vi "reserve.vi"(7 "LabVIEW Web Service Request":refnum<class "Web Request.lvclass">, 11 "context_id":string) -> (2 "reservation_id":string, 3 "load_url":string)   [LabVIEW 2013]
uses:
  <vilib>/wsapi/Web Request.lvclass
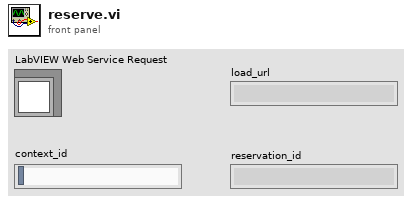
[diagram p1: front panel]
types:
  T1 = cluster{"laboratory_id":string, "username":string, "institution":string, "general_configuration_str":string, "particular_configurations":string, "request_payload":string, "user_properties":string, "locale":string, "back":string}
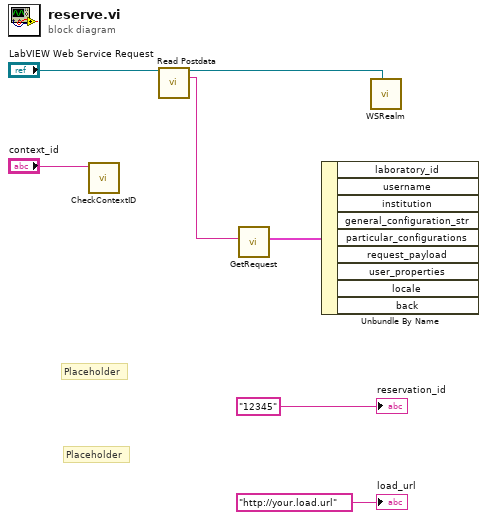
[diagram p0: block diagram]
diagram:
  # "Placeholder"
  # "Placeholder"
  n1 = call "CheckContextID.vi"("context_id"="context_id") -> ()  [unwired: 10 in, 1 out]
  n2 = call <vilib>:"Read Postdata.vi"("LabVIEW Web Service Request"="LabVIEW Web Service Request") -> ("LabVIEW Web Service Request out"=w5:refnum<class "Web Request.lvclass">, "postdata"=w4:string)  [unwired: 12 in, 1 out]
  n3 = call "GetRequest.vi"("JSON string"=w4) -> ("request"=w3:T1)  [unwired: 10 in]
  n4 = Unbundle By Name(w3) -> ()  [unwired: 9 out]
  n5 = call "WSRealm.vi"("LabVIEW Web Service Request"=w5) -> ()  [unwired: 11 in]
  "reservation_id" <- "12345"
  "load_url" <- "http://your.load.url" ("load_url")
